vi "Cavities_FPGA_v00.vi"() -> ()   [LabVIEW 2010]
doc: "Four cavities are controlled here:\n1) OPO A\n2) OPO B\n3) mode Cleaner\n4) Doubler\nThe output can either be Scanned, Locked, or Held."
uses:
  Strict Type Defs/Cavity Errors.ctl
  Strict Type Defs/Cavity Monitors.ctl
  Strict Type Defs/Zero Crossing.ctl
  Strict Type Defs/Control.ctl
  Strict Type Defs/PII individual.ctl
  Strict Type Defs/Safety First.ctl
  Strict Type Defs/Error Scale.ctl
  Strict Type Defs/Lock Thresh.ctl
  Strict Type Defs/Scope.ctl
  <vilib>/rvi/DataTransferAndStorage/Container/XNode/niFpgaContainer.xnode
  <vilib>/rvi/DataTransferAndStorage/Container/Common/niFpgaContainerMethod.ctl
  <vilib>/rvi/DataTransferAndStorage/Container/Common/niFpgaTransferTypeControl.ctl
  <vilib>/rvi/interface/RandomDataEmulation/nirviRandomDataFPGAFIFO.vi
  <vilib>/rvi/interface/RandomDataEmulation/niFpgaRandomDataHandleErrors.vi
panel:
  out "Unlocked?(T=yes)":T1
  in  "Lock Monitor":T2
  in  "Cavities Delay(uSec)":u32 caption="Count(uSec)"
  out "Lock Threshold":T3
  in  "Scope":T4={"Trigger Direction"=enum."plus-minus", "Delay"=0, "Aquisition Rate (Ticks)"=40, "Offset"=0, "Channel"=0, "Channel Selector"={"Channel 1"=0, "Channel 2"=4, "Channel 3"=8, "Channel 4"=8}} {"Channel Selector"."Channel 4" items=["Error Signal 1", "Error Signal 2", "Scan Trigger 1", "Scan Trigger 2", "DC Signal 1", "DC Signal 2", "PI Out 1", "PI Out 2"]; "Channel Selector"."Channel 3" items=["Error Signal 1", "Error Signal 2", "Scan Trigger 1", "Scan Trigger 2", "DC Signal 1", "DC Signal 2", "PI Out 1", "PI Out 2"]; "Channel Selector"."Channel 2" items=["Error Signal 1", "Error Signal 2", "Scan Trigger 1", "Scan Trigger 2", "DC Signal 1", "DC Signal 2", "PI Out 1", "PI Out 2"]; "Channel Selector"."Channel 1" items=["Error Signal 1", "Error Signal 2", "Scan Trigger 1", "Scan Trigger 2", "DC Signal 1", "DC Signal 2", "PI Out 1", "PI Out 2"]}
  in  "quit Control Loop":bool
  in  "Control":T5={"PII In 1"={"Lock"=FALSE, "Hold"=FALSE, "P Gain"=0, "P BS"=-5, "I Gain"=0, "I BS"=-10, "I2 G"=0, "I2 BS"=-26, "Scan Amp"=0, "Scan Off"=0, "Scan FS"=0, "SFS BS"=0, "I Max value"=10000, "I2 Max value"=10000, "Scope.Offset"=0, "Trigger Direction"=enum."either", "Scan-PII thresh"=0}, "PII In 2"={"Lock"=FALSE, "Hold"=FALSE, "P Gain"=0, "P BS"=-10, "I Gain"=0, "I BS"=-10, "I2 G"=0, "I2 BS"=-26, "Scan Amp"=0, "Scan Off"=0, "Scan FS"=0, "SFS BS"=0, "I Max value"=10000, "I2 Max value"=10000, "Scope.Offset"=0, "Trigger Direction"=enum."either", "Scan-PII thresh"=0}, "PII In 3"={"Lock"=FALSE, "Hold"=FALSE, "P Gain"=0, "P BS"=-10, "I Gain"=0, "I BS"=-10, "I2 G"=0, "I2 BS"=-26, "Scan Amp"=0, "Scan Off"=0, "Scan FS"=0, "SFS BS"=0, "I Max value"=10000, "I2 Max value"=10000, "Scope.Offset"=0, "Trigger Direction"=enum."either", "Scan-PII thresh"=0}, "PII In 4"={"Lock"=FALSE, "Hold"=FALSE, "P Gain"=0, "P BS"=-10, "I Gain"=0, "I BS"=-10, "I2 G"=0, "I2 BS"=-26, "Scan Amp"=0, "Scan Off"=0, "Scan FS"=0, "SFS BS"=0, "I Max value"=10000, "I2 Max value"=10000, "Scope.Offset"=0, "Trigger Direction"=enum."either", "Scan-PII thresh"=0}, "Safety First"={"lim reset"=FALSE, "no limit"=FALSE, "pos slew rate * dt"=10, "neg slew rate * dt"=-10, "Hold All"=FALSE, "Count(Ticks)"=0}, "Error scale"={"Pre-Offset"={"Pre-Offset 1"=2, "Pre-Offset 2"=0, "Pre-Offset 3"=0, "Pre-Offset 4"=0, "Pre-Offset 5"=2, "Pre-Offset 6"=0, "Pre-Offset 7"=0, "Pre-Offset 8"=0}, "Post-Offset "={"Offset 1"=0, "Offset 2"=300, "Offset 3"=0, "Offset 4"=0, "Offset 5"=0, "Offset 6"=0, "Offset 7"=0, "Offset 8"=0}, "Gains"={"Gain 1"=0, "Gain 2"=300, "Gain 3"=0, "Gain 4"=0, "Gain 5"=0, "Gain 6"=0, "Gain 7"=0, "Gain 8"=0}, "Polarity DC"={"False 1"=FALSE, "False 2"=FALSE, "False 3"=FALSE, "False 4"=FALSE, "DC x -1"=FALSE, "DC x -1 2"=FALSE, "DC x -1 3"=FALSE, "DC x -1 4"=FALSE}}, "Lock Thresh"={"OPO A"=2, "OPO B"=0, "MCC"=40, "Doubler"=0}, "Re-Scan Thresh"={"OPO A"=0, "OPO B"=0, "MCC"=0, "Doubler"=0}}
  in  "\"I too high?\"":T1
  in  "\"Outputs\"":T2
  out "Outputs":T10={"OPO A out"=-270, "OPO B out"=-1710, "MCC out"=880, "Doubler out"=570}
  in  "\"Trigger\"":T11
  out "Trigger":T11
  out "Cavity Monitors":T12
  out "Cavity Errors":T13={"OPO A"=0, "OPO B"=1800, "MCC"=0, "Doubler"=0}
  out "Control Loop count":i32=11285327
  out "Scope Full?":bool
  out "Scope loop count":i32=119818
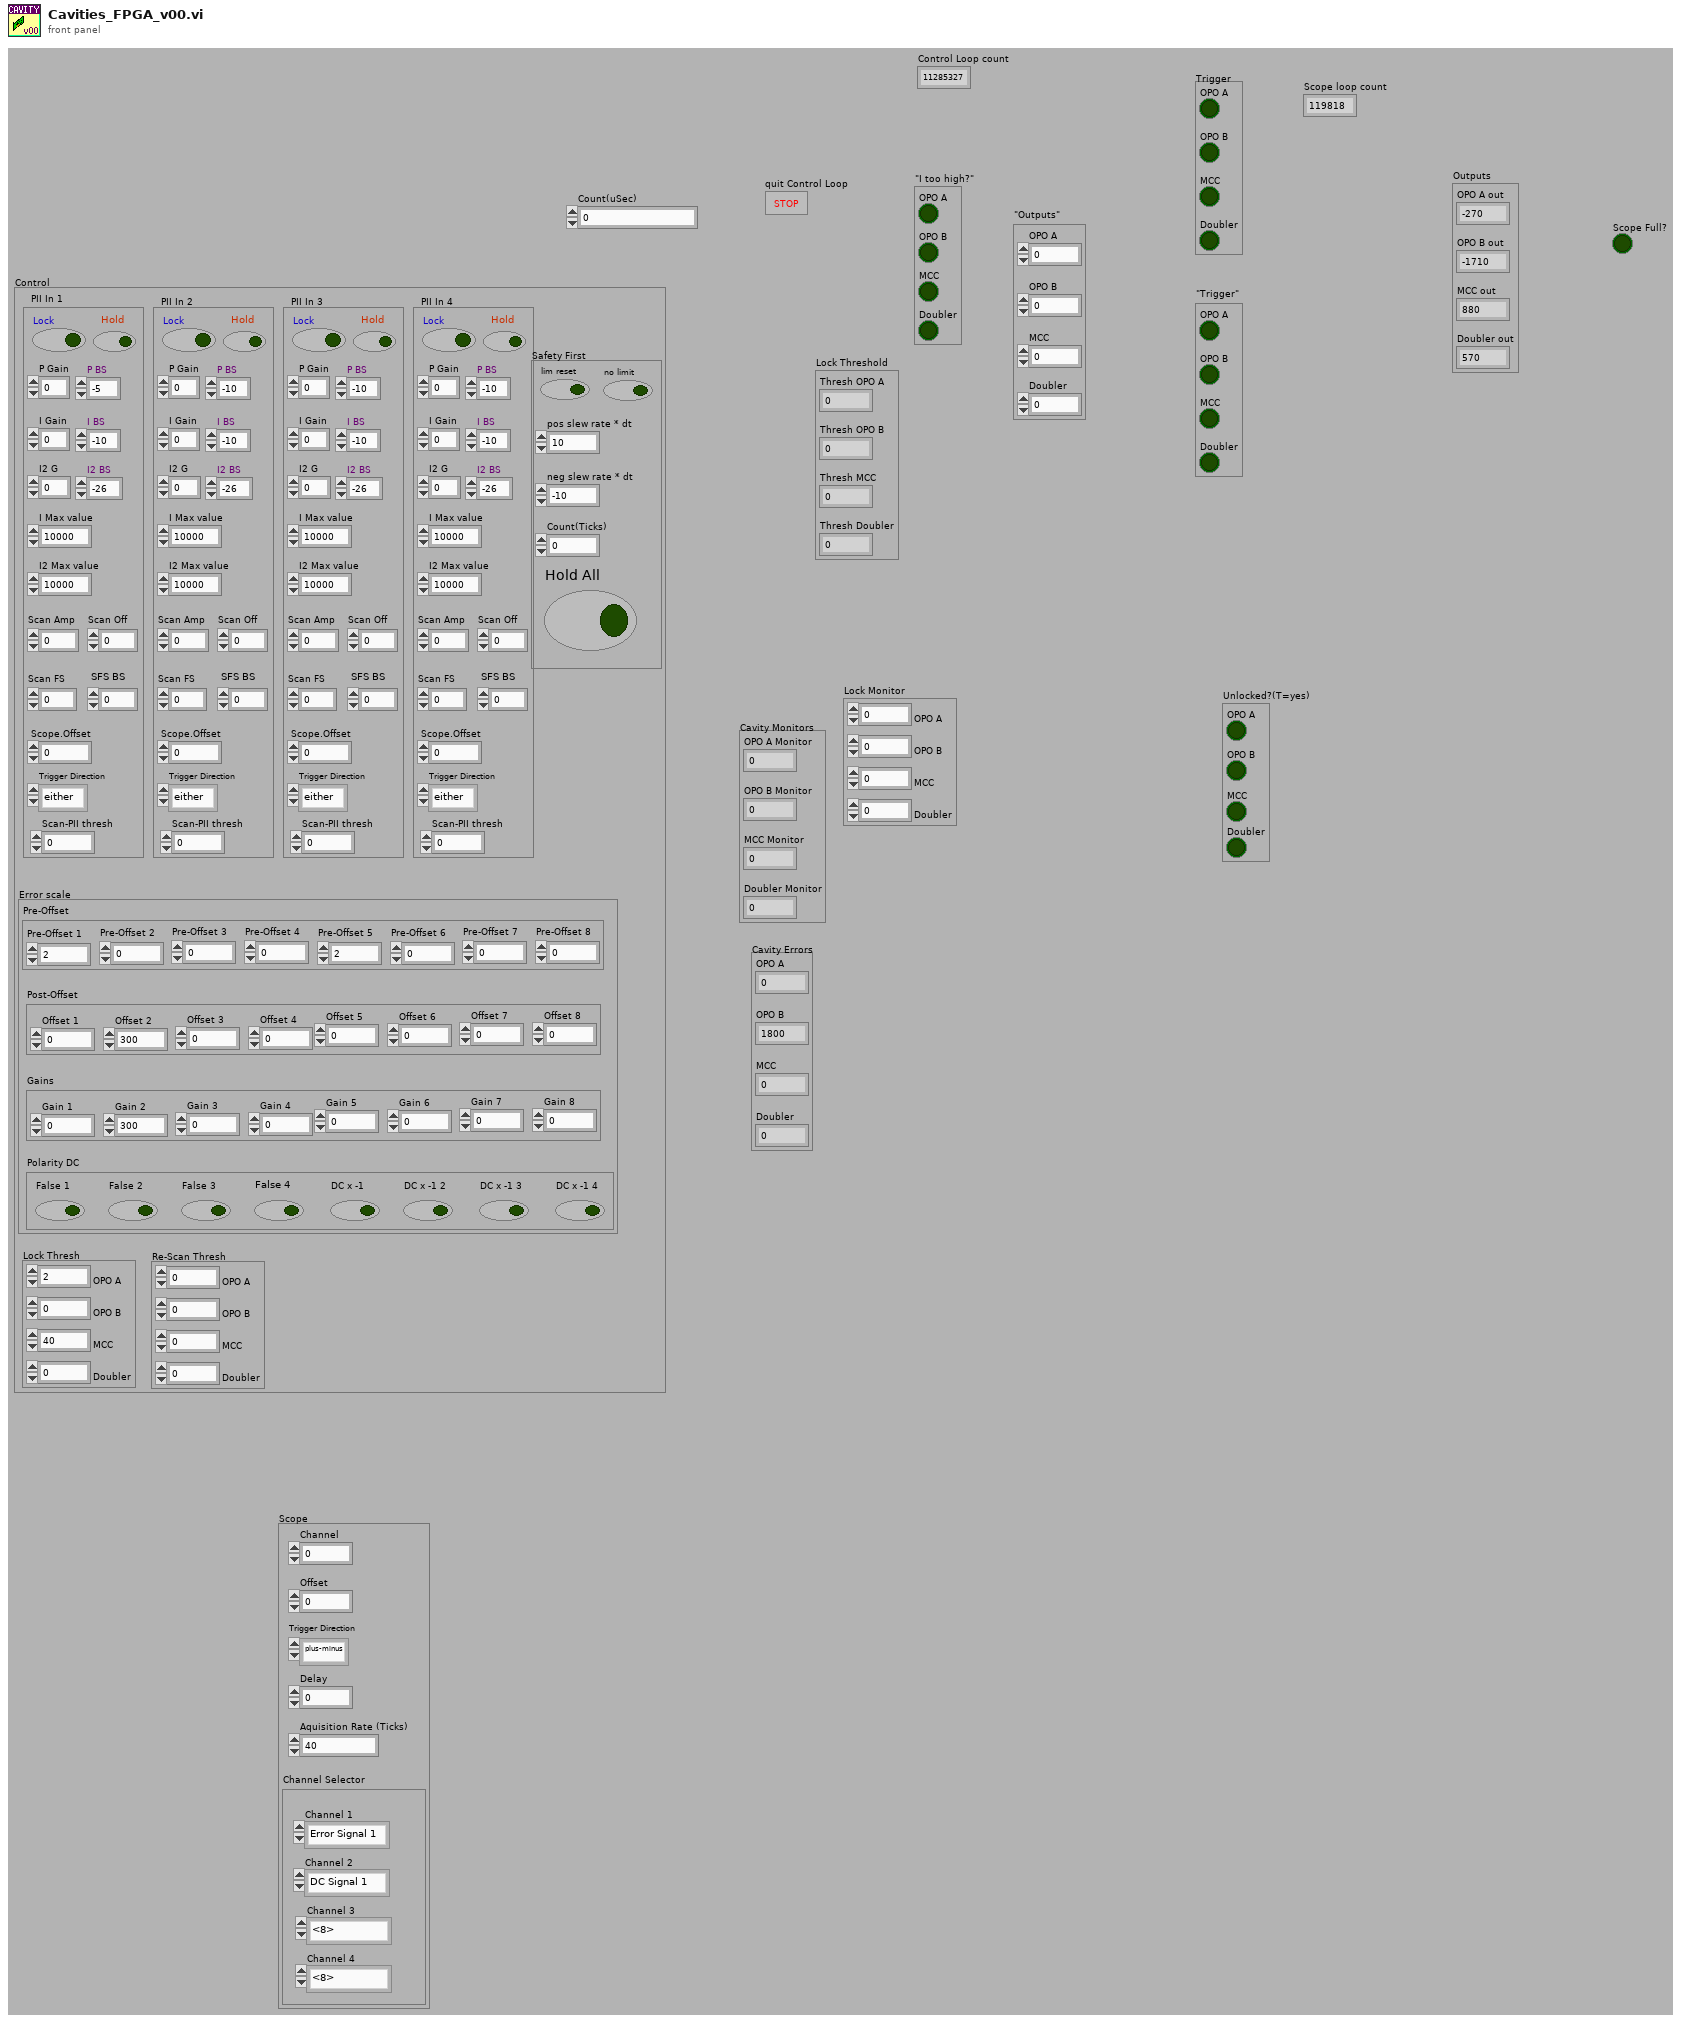
[diagram p1: front panel]
types:
  T1 = cluster{"OPO A":bool, "OPO B":bool, "MCC":bool, "Doubler":bool}
  T2 = cluster{"OPO A":i16, "OPO B":i16, "MCC":i16, "Doubler":i16}
  T3 = cluster{"Thresh OPO A ":i16, "Thresh OPO B":i16, "Thresh MCC":i16, "Thresh Doubler":i16}
  T4 = typedef "Scope.ctl" = cluster{"Trigger Direction":enum8{"either", "minus-plus", "plus-minus"}, "Delay":u32, "Aquisition Rate (Ticks)":u32, "Offset":i16, "Channel":i32, "Channel Selector":cluster{"Channel 1":i32, "Channel 2":i32, "Channel 3":i32, "Channel 4":i32}}
  T5 = typedef "Control.ctl" = cluster{"PII In 1":T6, "PII In 2":T6, "PII In 3":T6, "PII In 4":T6, "Safety First":T7, "Error scale":T8, "Lock Thresh":T9, "Re-Scan Thresh":T9}
  T6 = typedef "PII individual.ctl" = cluster{"Lock":bool, "Hold":bool, "P Gain":i32, "P BS":i16, "I Gain":i32, "I BS":i16, "I2 G":i32, "I2 BS":i16, "Scan Amp":i16, "Scan Off":i16, "Scan FS":u16, "SFS BS":i16, "I Max value":i32, "I2 Max value":i32, "Scope.Offset":i16, "Trigger Direction":enum8{"either", "minus-plus", "plus-minus"}, "Scan-PII thresh":i16}
  T7 = typedef "Safety First.ctl" = cluster{"lim reset":bool, "no limit":bool, "pos slew rate * dt":i16, "neg slew rate * dt":i16, "Hold All":bool, "Count(Ticks)":u32}
  T8 = typedef "Error Scale.ctl" = cluster{"Pre-Offset":cluster{"Pre-Offset 1":i16, "Pre-Offset 2":i16, "Pre-Offset 3":i16, "Pre-Offset 4":i16, "Pre-Offset 5":i16, "Pre-Offset 6":i16, "Pre-Offset 7":i16, "Pre-Offset 8":i16}, "Post-Offset ":cluster{"Offset 1":i16, "Offset 2":i16, "Offset 3":i16, "Offset 4":i16, "Offset 5":i16, "Offset 6":i16, "Offset 7":i16, "Offset 8":i16}, "Gains":cluster{"Gain 1":i16, "Gain 2":i16, "Gain 3":i16, "Gain 4":i16, "Gain 5":i16, "Gain 6":i16, "Gain 7":i16, "Gain 8":i16}, "Polarity DC":cluster{"False 1":bool, "False 2":bool, "False 3":bool, "False 4":bool, "DC x -1":bool, "DC x -1 2":bool, "DC x -1 3":bool, "DC x -1 4":bool}}
  T9 = typedef "Lock Thresh.ctl" = cluster{"OPO A":i16, "OPO B":i16, "MCC":i16, "Doubler":i16}
  T10 = cluster{"OPO A out":i16, "OPO B out":i16, "MCC out":i16, "Doubler out":i16}
  T11 = typedef "Zero Crossing.ctl" = cluster{"OPO A":bool, "OPO B":bool, "MCC":bool, "Doubler":bool}
  T12 = typedef "Cavity Monitors.ctl" = cluster{"OPO A Monitor":i16, "OPO B Monitor":i16, "MCC Monitor":i16, "Doubler Monitor":i16}
  T13 = typedef "Cavity Errors.ctl" = cluster{"OPO A":i16, "OPO B":i16, "MCC":i16, "Doubler":i16}
  T14 = typedef "niFpgaContainerMethod.ctl" = enum16{"<none>", "write", "read", "clear", "getNumberOfElementsToWrite", "getNumberOfElementsToRead", "enable", "disable", "flushAndDisable", "getStreamState", "readA", "readB", "dramWrite", "dramWriteWithByteEnables", "dramRequestData", "dramRetrieveData"}
  T15 = typedef "niFpgaTransferTypeControl.ctl" = enum16{"Target-Scoped", "Host to Target - DMA", "Target to Host - DMA", "Peer to Peer Reader", "Peer to Peer Writer", "Bidirectional"}
  T16 = typedef "Signals.ctl" = cluster{"Cavity Errors":T13, "Cavity Monitors":T12, "Lock Thresh":T9, "Re-Scan Thresh":T9, "PII In 1":T6, "PII In 2":T6, "PII In 3":T6, "PII In 4":T6, "Safety First":T7}
  T17 = typedef "Control Cavity Cluster.ctl" = cluster{"Control A":T6, "Control B":T6, "Control MCC":T6, "Control Doubler":T6, "Lock Point?":T18, "Re-scan?":T19, "Cavity Errors":T13, "Max":T20, "Min":T21, "Lock Threshold":cluster{"Thresh OPO A ":i16, "Thresh OPO B":i16, "Thresh MCC":i16, "Thresh Doubler":i16}, "Re-Scan Threshold":cluster{"Thresh OPO A ":i16, "Thresh OPO B":i16, "Thresh MCC":i16, "Thresh Doubler":i16}, "State (-1)":cluster{"OPO A":enum16{"Safe", "Hold", "Scan", "Lock"}, "OPO B":enum16{"Safe", "Hold", "Scan", "Lock"}, "MCC":enum16{"Safe", "Hold", "Scan", "Lock"}, "Doubler":enum16{"Safe", "Hold", "Scan", "Lock"}}, "Lock pressed? (-1)":cluster{"OPO A":bool, "OPO B":bool, "MCC":bool, "Doubler":bool}, "Safety First":T7}
  T18 = typedef "Lock Point.ctl" = cluster{"OPO A":bool, "OPO B":bool, "MCC":bool, "Doubler":bool}
  T19 = typedef "Re-Scan.ctl" = cluster{"OPO A":bool, "OPO B":bool, "MCC":bool, "Doubler":bool}
  T20 = typedef "Max.ctl" = cluster{"Max OPO A":i16, "Max OPO B":i16, "Max MCC":i16, "Max Doubler":i16}
  T21 = typedef "Min.ctl" = cluster{"Min OPO A":i16, "Min OPO B":i16, "Min MCC":i16, "Min Doubler":i16}
  T22 = typedef "PII Scan State.ctl" = cluster{"Control A":T6, "Control B":T6, "Control MCC":T6, "Control Doubler":T6, "Cavity Errors":T13, "State":cluster{"OPO A":enum16{"Safe", "Hold", "Scan", "Lock"}, "OPO B":enum16{"Safe", "Hold", "Scan", "Lock"}, "MCC":enum16{"Safe", "Hold", "Scan", "Lock"}, "Doubler":enum16{"Safe", "Hold", "Scan", "Lock"}}}
  T23 = typedef "MaxMin.ctl" = cluster{"State":cluster{"OPO A":enum16{"Safe", "Hold", "Scan", "Lock"}, "OPO B":enum16{"Safe", "Hold", "Scan", "Lock"}, "MCC":enum16{"Safe", "Hold", "Scan", "Lock"}, "Doubler":enum16{"Safe", "Hold", "Scan", "Lock"}}, "Reset MaxMin?":cluster{"OPO A":bool, "OPO B":bool, "MCC":bool, "Doubler":bool}, "Max":T20, "Min":T21, "Lock pressed?":cluster{"OPO A":bool, "OPO B":bool, "MCC":bool, "Doubler":bool}, "Safety First":T7}
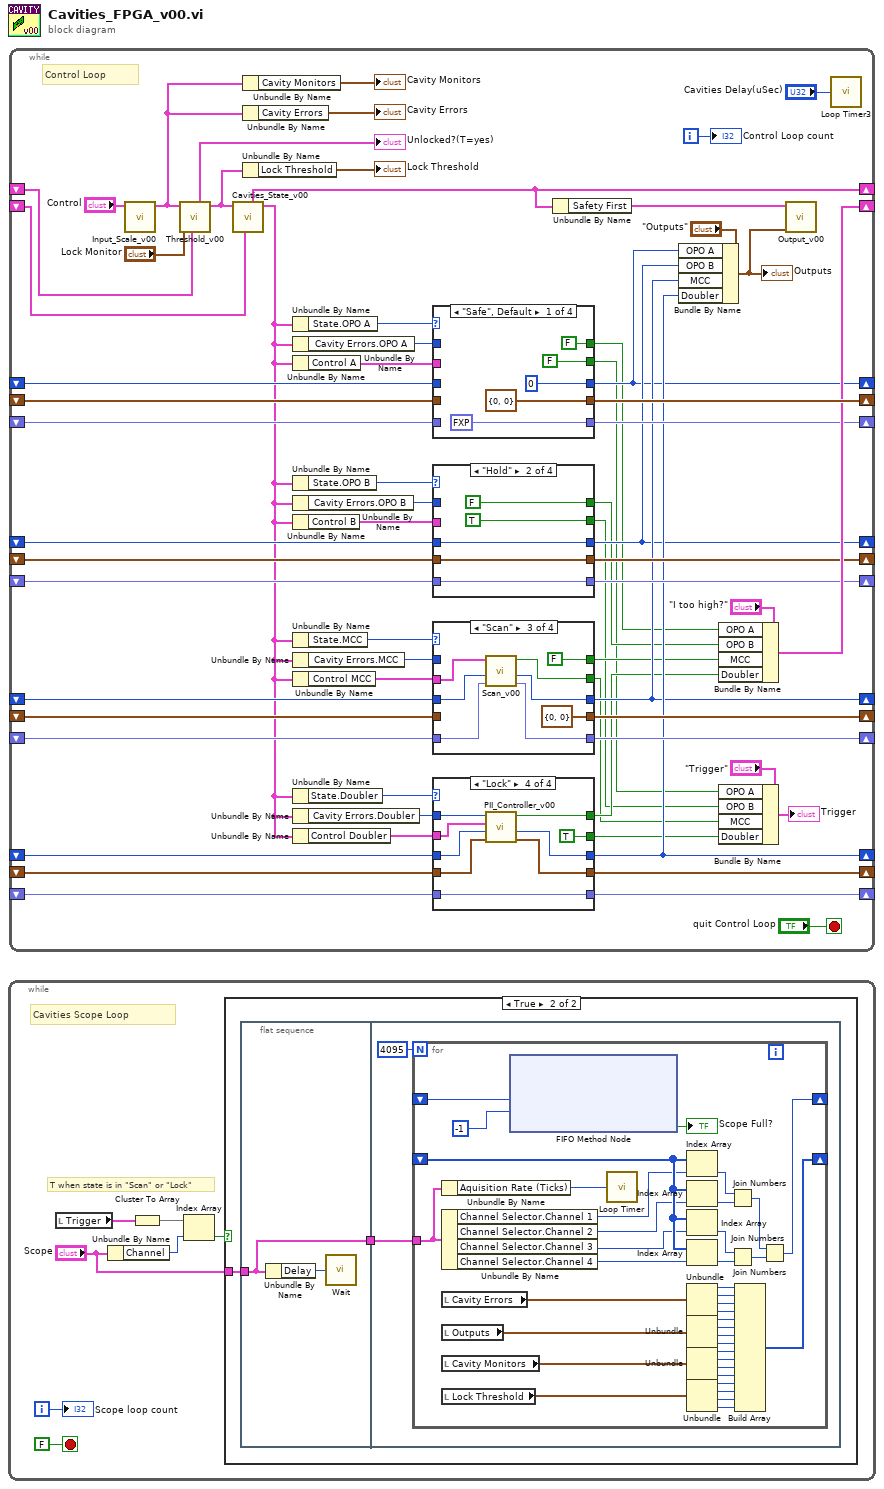
[diagram p0: block diagram]
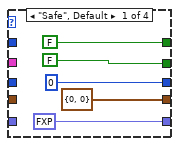
[diagram p3: hidden frame]
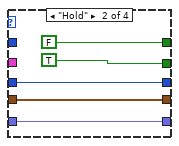
[diagram p4: hidden frame]
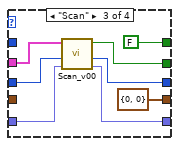
[diagram p5: hidden frame]
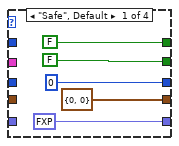
[diagram p6: hidden frame]
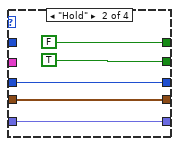
[diagram p7: hidden frame]
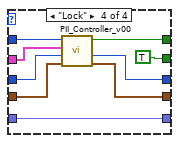
[diagram p8: hidden frame]
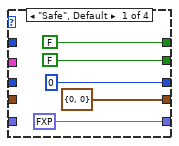
[diagram p9: hidden frame]
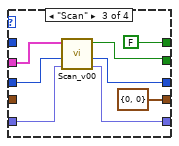
[diagram p10: hidden frame]
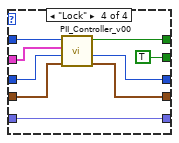
[diagram p11: hidden frame]
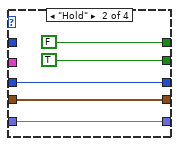
[diagram p12: hidden frame]
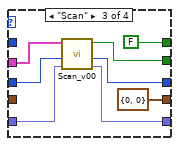
[diagram p13: hidden frame]
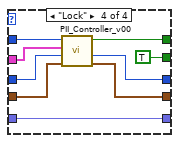
[diagram p14: hidden frame]
diagram:
  n1 = while {
    i -> [w4]
    stop <- FALSE ("stop") stop-if-true
    # "Cavities Scope Loop"
    # "T when state is in \"Scan\" or \"Lock\""
    n2 = local read "Trigger"() -> (w2:T11)
    n3 = Unbundle By Name("Scope") -> ("Channel"=w5:i32)
    n4 = Cluster To Array(cluster=w2) -> (array=w6:bool[])
    n5 = Index Array(array=w6, index=w5) -> (element=w3:bool)
    n6 = case shown="True" w3 {
      tunnel: "Scope" -> [_ w9]
      frame False {
      }
      frame True {
        n7 = flat-sequence {
          tunnel: w9 -> [w10]
          tunnel: [w10] -> w8
          tunnel: w8 -> [w12]
          frame #0 {
            n8 = Unbundle By Name(w10) -> ("Delay"=w11:u32)
            n9 = call "Wait"("Count(Ticks)"=w11) -> ()  [unwired: 1 out]
          }
          frame #1 {
            n10 = for {
              N: 4095 -> [_]
              tunnel: w12 -> [w50]
              shift-right: [w29] -> _
              shift-left: _ -> [w28]
              shift-right: [w24] -> _
              shift-left: _ -> [w23]
              n11 = Unbundle By Name(w50) -> ("Aquisition Rate (Ticks)"=w51:u32)
              n12 = Unbundle By Name(w50) -> ("Channel Selector.Channel 1"=w25:i32, "Channel Selector.Channel 2"=w26:i32, "Channel Selector.Channel 3"=w16:i32, "Channel Selector.Channel 4"=w27:i32)
              n13 = local read "Cavity Errors"() -> (w49:T13)
              n14 = local read "Outputs"() -> (w48:T10)
              n15 = local read "Cavity Monitors"() -> (w47:T12)
              n16 = local read "Lock Threshold"() -> (w14:T3)
              n17 = xnode ("FIFO Method Node")("Element"=w23, "Timeout"=-1) -> ("Timed Out?"=→"Scope Full?":bool)  [unwired: 1 in, 1 out]
              n18 = call "Loop Timer"("Count(uSec)"=w51) -> ()  [unwired: 1 out]
              n19 = Index Array(array=w28, index=w25) -> (element=w31:i16)
              n20 = Index Array(array=w28, index=w26) -> (element=w30:i16)
              n21 = Index Array(array=w28, index=w16) -> (element=w15:i16)
              n22 = Index Array(array=w28, index=w27) -> (element=w32:i16)
              n23 = Unbundle(w49) -> ("OPO A"=w46:i16, "OPO B"=w45:i16, "MCC"=w44:i16, "Doubler"=w43:i16)
              n24 = Unbundle(w48) -> ("OPO A out"=w42:i16, "OPO B out"=w41:i16, "MCC out"=w40:i16, "Doubler out"=w39:i16)
              n25 = Unbundle(w47) -> ("OPO A Monitor"=w38:i16, "OPO B Monitor"=w37:i16, "MCC Monitor"=w36:i16, "Doubler Monitor"=w35:i16)
              n26 = Unbundle(w14) -> ("Thresh OPO A"=w18:i16, "Thresh OPO B"=w19:i16, "Thresh MCC"=w20:i16, "Thresh Doubler"=w21:i16)
              n27 = Join Numbers(hi=w31, lo=w30) -> ((hi.lo)=w34:u32)
              n28 = Join Numbers(hi=w15, lo=w32) -> ((hi.lo)=w33:u32)
              n29 = Build Array(w46, w45, w44, w43, w42, w41, w40, w39, w38, w37, w36, w35, w18, w19, w20, w21) -> (w29:i16[])
              n30 = Join Numbers(hi=w34, lo=w33) -> ((hi.lo)=w24:u64)
            }
          }
        }
      }
    }
    "Scope loop count" <- w4
  }
  n31 = while {
    shift-right: [w144] -> _
    shift-left: _ -> [w142]
    shift-right: [w141] -> _
    shift-left: _ -> [w80]
    shift-right: [w110] -> _
    shift-left: _ -> [w143]
    shift-right: [w138] -> _
    shift-left: _ -> [w137]
    shift-right: [w116] -> _
    shift-left: _ -> [w81]
    shift-right: [w127] -> _
    shift-left: _ -> [w129]
    shift-right: [w111] -> _
    shift-left: _ -> [w128]
    shift-right: [w130] -> _
    shift-left: _ -> [w131]
    shift-right: [w126] -> _
    shift-left: _ -> [w124]
    shift-right: [w112] -> _
    shift-left: _ -> [w125]
    shift-right: [w123] -> _
    shift-left: _ -> [w122]
    shift-right: [w117] -> _
    shift-left: _ -> [w119]
    shift-right: [w113] -> _
    shift-left: _ -> [w118]
    shift-right: [w120] -> _
    shift-left: _ -> [w121]
    i -> [w134]
    stop <- "quit Control Loop" stop-if-true
    # "Control Loop"
    n32 = call "Input_Scale_v00.vi"("Control"="Control") -> ("Signals"=w98:T16)  [unwired: 10 in]
    n33 = call "Threshold_v00.vi"("MaxMin"=w81, "Lock Monitor"="Lock Monitor", "Signals"=w98) -> ("Control Cavity Cluster"=w102:T17, "Unlocked?(T=yes)"=→"Unlocked?(T=yes)":T1)  [unwired: 7 in]
    n34 = call "Cavities_State_v00.vi"("\"I too high?\""=w80, "Control Cavity Cluster"=w102) -> ("PII Scan State Errors"=w82:T22, "MaxMin"=w116:T23)  [unwired: 8 in]
    n35 = Unbundle By Name(w98) -> ("Cavity Monitors"=→"Cavity Monitors":T12)
    n36 = Unbundle By Name(w98) -> ("Cavity Errors"=→"Cavity Errors":T13)
    n37 = Unbundle By Name(w102) -> ("Lock Threshold"=→"Lock Threshold":T3)
    n38 = Unbundle By Name(w82) -> ("State.OPO A"=w132:enum16{"Safe", "Hold", "Scan", "Lock"})
    n39 = Unbundle By Name(w82) -> ("Cavity Errors.OPO A"=w92:i16)
    n40 = Unbundle By Name(w82) -> ("Control A"=w93:T6)
    n41 = Unbundle By Name(w82) -> ("State.OPO B"=w90:enum16{"Safe", "Hold", "Scan", "Lock"})
    n42 = Unbundle By Name(w82) -> ("Cavity Errors.OPO B"=w91:i16)
    n43 = Unbundle By Name(w82) -> ("Control B"=w89:T6)
    n44 = Unbundle By Name(w82) -> ("State.MCC"=w88:enum16{"Safe", "Hold", "Scan", "Lock"})
    n45 = Unbundle By Name(w82) -> ("Cavity Errors.MCC"=w87:i16)
    n46 = Unbundle By Name(w82) -> ("Control MCC"=w86:T6)
    n47 = Unbundle By Name(w82) -> ("State.Doubler"=w85:enum16{"Safe", "Hold", "Scan", "Lock"})
    n48 = Unbundle By Name(w82) -> ("Cavity Errors.Doubler"=w84:i16)
    n49 = Unbundle By Name(w82) -> ("Control Doubler"=w83:T6)
    n50 = case shown="\"Safe\", Default" w132 {
      tunnel: w92 -> [_ _ _ w253]
      tunnel: [cluster{"I Cavity":i32, "I2 Cavity":i32} {"I Cavity"=0, "I2 Cavity"=0} ("Integrator") w234 cluster{"I Cavity":i32, "I2 Cavity":i32} {"I Cavity"=0, "I2 Cavity"=0} ("Integrator") w249] -> w144
      tunnel: [FALSE ("I too high? (F=No)") FALSE ("I too high? (F=No)") FALSE ("I too high? (F=No)") w252] -> w109
      tunnel: w93 -> [_ _ w243 w250]
      tunnel: [i16 0 ("PII out") w235 w242 w246] -> w110
      tunnel: w143 -> [_ w235 w239 w247]
      tunnel: w142 -> [_ w234 _ w251]
      tunnel: [fxp<+,33,17> 0.0 ("Scan") w233 w241 w245] -> w138
      tunnel: w137 -> [_ w233 w240 w245]
      tunnel: [FALSE ("Zero Crossing") TRUE ("Zero Crossing") w238 TRUE ("Zero Crossing")] -> w105
      frame "Safe", Default {
      }
      frame "Hold" {
      }
      frame "Scan" {
        n51 = call "Scan_v00.vi"("Scan (-1)"=w240, "Scan out (-1)"=w239, "Control Cavity"=w243) -> ("Scan"=w241:fxp<+,33,17>, "Scan out"=w242:i16, "Zero Crossing"=w238:bool)  [unwired: 6 in]
      }
      frame "Lock" {
        n52 = call "PII_Controller_v00.vi"("Integrator (-1)"=w251, "PII out (-1)"=w247, "Control Cavity"=w250, "OPO A Error"=w253) -> ("Integrator"=w249:cluster{"I Cavity":i32, "I2 Cavity":i32}, "PII out"=w246:i16, "I too high?"=w252:bool)  [unwired: 5 in]
      }
    }
    n53 = case shown="\"Hold\"" w90 {
      tunnel: w91 -> [_ _ _ w226]
      tunnel: [cluster{"I Cavity":i32, "I2 Cavity":i32} {"I Cavity"=0, "I2 Cavity"=0} ("Integrator") w207 cluster{"I Cavity":i32, "I2 Cavity":i32} {"I Cavity"=0, "I2 Cavity"=0} ("Integrator") w222] -> w127
      tunnel: [FALSE ("I too high? (F=No)") FALSE ("I too high? (F=No)") FALSE ("I too high? (F=No)") w225] -> w108
      tunnel: w89 -> [_ _ w216 w223]
      tunnel: [i16 0 ("PII out") w208 w215 w220] -> w111
      tunnel: w128 -> [_ w208 w212 w221]
      tunnel: w129 -> [_ w207 _ w224]
      tunnel: [fxp<+,33,17> 0.0 ("Scan") w206 w214 w219] -> w130
      tunnel: w131 -> [_ w206 w213 w219]
      tunnel: [FALSE ("Zero Crossing") TRUE ("Zero Crossing") w210 TRUE ("Zero Crossing")] -> w97
      frame "Safe", Default {
      }
      frame "Hold" {
      }
      frame "Scan" {
        n54 = call "Scan_v00.vi"("Scan (-1)"=w213, "Scan out (-1)"=w212, "Control Cavity"=w216) -> ("Scan"=w214:fxp<+,33,17>, "Scan out"=w215:i16, "Zero Crossing"=w210:bool)  [unwired: 6 in]
      }
      frame "Lock" {
        n55 = call "PII_Controller_v00.vi"("Integrator (-1)"=w224, "PII out (-1)"=w221, "Control Cavity"=w223, "OPO A Error"=w226) -> ("Integrator"=w222:cluster{"I Cavity":i32, "I2 Cavity":i32}, "PII out"=w220:i16, "I too high?"=w225:bool)  [unwired: 5 in]
      }
    }
    n56 = case shown="\"Scan\"" w88 {
      tunnel: w87 -> [_ _ _ w199]
      tunnel: [cluster{"I Cavity":i32, "I2 Cavity":i32} {"I Cavity"=0, "I2 Cavity"=0} ("Integrator") w180 cluster{"I Cavity":i32, "I2 Cavity":i32} {"I Cavity"=0, "I2 Cavity"=0} ("Integrator") w195] -> w126
      tunnel: [FALSE ("I too high? (F=No)") FALSE ("I too high? (F=No)") FALSE ("I too high? (F=No)") w198] -> w107
      tunnel: w86 -> [_ _ w189 w196]
      tunnel: [i16 0 ("PII out") w181 w188 w192] -> w112
      tunnel: w125 -> [_ w181 w185 w193]
      tunnel: w124 -> [_ w180 _ w197]
      tunnel: [fxp<+,33,17> 0.0 ("Scan") w179 w187 w191] -> w123
      tunnel: w122 -> [_ w179 w186 w191]
      tunnel: [FALSE ("Zero Crossing") TRUE ("Zero Crossing") w184 TRUE ("Zero Crossing")] -> w104
      frame "Safe", Default {
      }
      frame "Hold" {
      }
      frame "Scan" {
        n57 = call "Scan_v00.vi"("Scan (-1)"=w186, "Scan out (-1)"=w185, "Control Cavity"=w189) -> ("Scan"=w187:fxp<+,33,17>, "Scan out"=w188:i16, "Zero Crossing"=w184:bool)  [unwired: 6 in]
      }
      frame "Lock" {
        n58 = call "PII_Controller_v00.vi"("Integrator (-1)"=w197, "PII out (-1)"=w193, "Control Cavity"=w196, "OPO A Error"=w199) -> ("Integrator"=w195:cluster{"I Cavity":i32, "I2 Cavity":i32}, "PII out"=w192:i16, "I too high?"=w198:bool)  [unwired: 5 in]
      }
    }
    n59 = case shown="\"Lock\"" w85 {
      tunnel: w84 -> [_ _ _ w172]
      tunnel: [cluster{"I Cavity":i32, "I2 Cavity":i32} {"I Cavity"=0, "I2 Cavity"=0} ("Integrator") w153 cluster{"I Cavity":i32, "I2 Cavity":i32} {"I Cavity"=0, "I2 Cavity"=0} ("Integrator") w168] -> w117
      tunnel: [FALSE ("I too high? (F=No)") FALSE ("I too high? (F=No)") FALSE ("I too high? (F=No)") w171] -> w106
      tunnel: w83 -> [_ _ w162 w169]
      tunnel: [i16 0 ("PII out") w154 w161 w165] -> w113
      tunnel: w118 -> [_ w154 w158 w166]
      tunnel: w119 -> [_ w153 _ w170]
      tunnel: [fxp<+,33,17> 0.0 ("Scan") w152 w160 w164] -> w120
      tunnel: w121 -> [_ w152 w159 w164]
      tunnel: [FALSE ("Zero Crossing") TRUE ("Zero Crossing") w157 TRUE ("Zero Crossing")] -> w103
      frame "Safe", Default {
      }
      frame "Hold" {
      }
      frame "Scan" {
        n60 = call "Scan_v00.vi"("Scan (-1)"=w159, "Scan out (-1)"=w158, "Control Cavity"=w162) -> ("Scan"=w160:fxp<+,33,17>, "Scan out"=w161:i16, "Zero Crossing"=w157:bool)  [unwired: 6 in]
      }
      frame "Lock" {
        n61 = call "PII_Controller_v00.vi"("Integrator (-1)"=w170, "PII out (-1)"=w166, "Control Cavity"=w169, "OPO A Error"=w172) -> ("Integrator"=w168:cluster{"I Cavity":i32, "I2 Cavity":i32}, "PII out"=w165:i16, "I too high?"=w171:bool)  [unwired: 5 in]
      }
    }
    n62 = Unbundle By Name(w116) -> ("Safety First"=w115:T7)
    n63 = Bundle By Name(cluster="\"Outputs\"", "OPO A"=w110, "OPO B"=w111, "MCC"=w112, "Doubler"=w113) -> (w114:T2)
    "Outputs" <- w114
    n64 = Bundle By Name(cluster="\"I too high?\"", "OPO A"=w109, "OPO B"=w108, "MCC"=w107, "Doubler"=w106) -> (w141:T1)
    n65 = Bundle By Name(cluster="\"Trigger\"", "OPO A"=w105, "OPO B"=w97, "MCC"=w104, "Doubler"=w103) -> (→"Trigger":T11)
    n66 = call "Output_v00.vi"("Outputs"=w114, "Safety First"=w115) -> ()  [unwired: 10 in]
    n67 = call "Loop Timer3"("Count(uSec)"="Cavities Delay(uSec)") -> ()  [unwired: 1 out]
    "Control Loop count" <- w134
  }
